vi "Write Facing.vi"(2 "error in (no error)":errorcluster, 3 "Facing":dbl, 4 "Sensor.lvclass":refnum<class "Sensor.lvclass">) -> (0 "error out":errorcluster, 1 "Sensor.lvclass":refnum<class "Sensor.lvclass">)   [LabVIEW 2015, in "Sensor.lvclass"]
uses:
  Sensor.lvclass
  Sensor.lvclass/Sensor.ctl
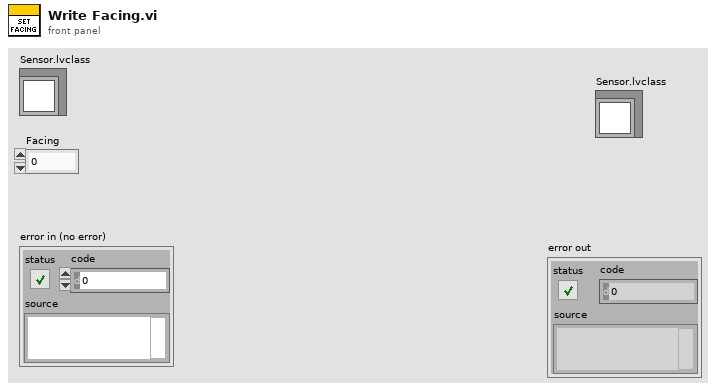
[diagram p1: front panel]
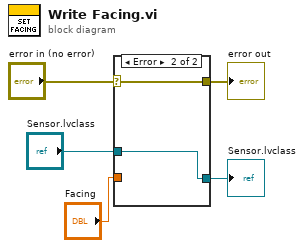
[diagram p0: block diagram]
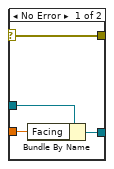
[diagram p2: hidden frame]
diagram:
  n1 = case shown="Error" "error in (no error)" {
    selector: "error in (no error)" -> [w9 w10]
    tunnel: [w9 w10] -> w4
    tunnel: "Facing" -> [w8 _]
    tunnel: "Sensor.lvclass" -> [w7 w11]
    tunnel: [w6 w11] -> w1
    frame No Error {
      n2 = Bundle By Name(cluster=w7, "Facing"=w8) -> (w6:refnum<class "Sensor.lvclass">)
    }
    frame Error {
    }
  }
  "error out" <- w4
  "Sensor.lvclass" <- w1
